vi "Min Buffer Size Test.vi"(7 "Fs (Hz)":dbl, 9 "Npts":i32) -> (15 "error out":errorcluster)   [LabVIEW 2015]
uses:
  <vilib>/DAQmx/write.llb/DAQmx Write (Digital Wfm 1Chan NSamp).vi
  <vilib>/DAQmx/write.llb/DAQmx Write (Analog 1D DBL 1Chan NSamp).vi
  <vilib>/DAQmx/create/channels.llb/DAQmx Create Channel (AO-Voltage-Basic).vi
  <vilib>/DAQmx/configure/timing.llb/DAQmx Timing (Sample Clock).vi
  <vilib>/DAQmx/miscellaneous.llb/DAQmx Fill In Error Info.vi
  <vilib>/DAQmx/create/channels.llb/DAQmx Create Channel (DO-Digital Output).vi
  <vilib>/Waveform/DWDTOps.llb/DWDT Boolean Array to Digital.vi
  <vilib>/Waveform/DWDTOps.llb/DWDT Uncompress Digital.vi
  <resource>/objmgr/daqmx.rc
panel:
  in  "stop":bool
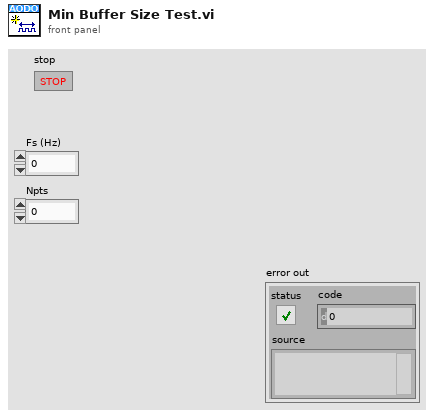
[diagram p1: front panel]
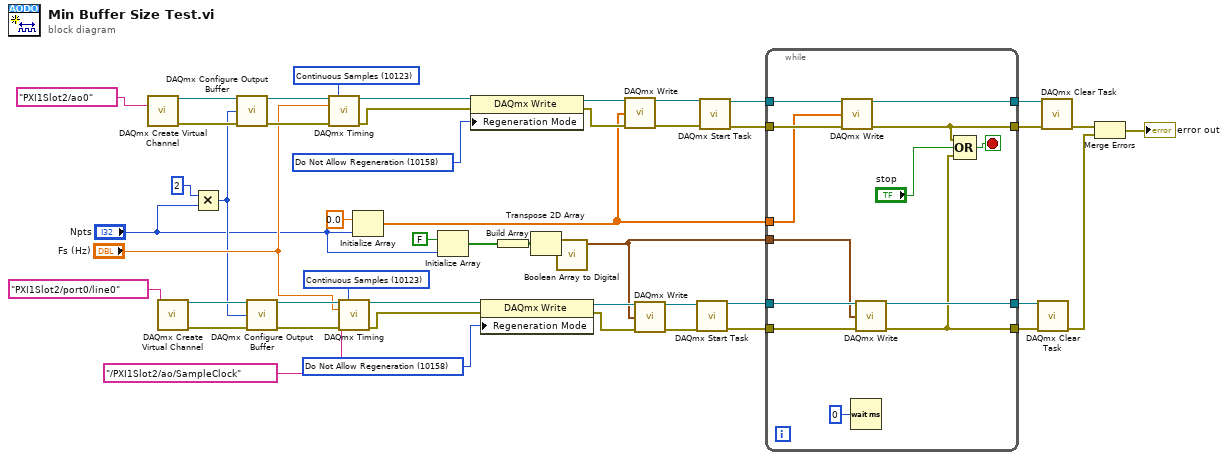
[diagram p0: block diagram]
diagram:
  w23 = 10158 items=["Allow Regeneration"=10097, "Do Not Allow Regeneration"=10158] ("RegenMode")
  w24 = 10123 items=["Finite Samples"=10178, "Continuous Samples"=10123, "Hardware Timed Single Point"=12522] ("sample mode")
  w43 = 10158 items=["Allow Regeneration"=10097, "Do Not Allow Regeneration"=10158] ("RegenMode")
  w44 = 10123 items=["Finite Samples"=10178, "Continuous Samples"=10123, "Hardware Timed Single Point"=12522] ("sample mode")
  n1 = call-poly <vilib>:"DAQmx Create Virtual Channel.vi"("physical channels"=tag "PXI1Slot2/ao0") -> ("task out"=w41:refnum<k21>, "error out"=w42:errorcluster)  [unwired: 13 in]
  n2 = call-poly <vilib>:"DAQmx Create Virtual Channel.vi"("lines"=tag "PXI1Slot2/port0/line0") -> ("task out"=w21:refnum<k21>, "error out"=w22:errorcluster)  [unwired: 13 in]
  n3 = Multiply(x=2 ("y"), y="Npts") -> (x*y=w15:i32)
  n4 = call <vilib>:"DAQmx Configure Output Buffer.vi"("task/channels in"=w41, "buffer size (in samples per channel)"=w15, "error in"=w42) -> ("task out"=w46:refnum<k21>, "error out"=w45:errorcluster)  [unwired: 11 in]
  n5 = call <vilib>:"DAQmx Configure Output Buffer.vi"("task/channels in"=w21, "buffer size (in samples per channel)"=w15, "error in"=w22) -> ("task out"=w26:refnum<k21>, "error out"=w25:errorcluster)  [unwired: 11 in]
  n6 = call-poly <vilib>:"DAQmx Timing.vi"("task/channels in"=w46, "sample mode"=w44, "rate"="Fs (Hz)", "error in"=w45) -> ("task out"=w48:refnum<k21>, "error out"=w47:errorcluster)  [unwired: 10 in]
  n7 = call-poly <vilib>:"DAQmx Timing.vi"("task/channels in"=w26, "sample mode"=w24, "rate"="Fs (Hz)", "source"=tag "/PXI1Slot2/ao/SampleClock", "error in"=w25) -> ("task out"=w28:refnum<k21>, "error out"=w27:errorcluster)  [unwired: 9 in]
  n8 = Initialize Array(0.0 ("element"), "Npts") -> (w32:dbl[])
  n9 = Initialize Array(FALSE, "Npts") -> (w12:bool[])
  n10 = property class="DAQmx Write"(reference=w48, error in=w47, "Regeneration Mode"=w43) -> (reference out=w39:refnum<k21>, error out=w38:errorcluster)
  n11 = property class="DAQmx Write"(reference=w28, error in=w27, "Regeneration Mode"=w23) -> (reference out=w20:refnum<k21>, error out=w19:errorcluster)
  n12 = Build Array(w12) -> (w11:bool[][])
  n13 = Transpose 2D Array(2D array=w11) -> (transposed array=w1:bool[][])
  n14 = call-poly <vilib>:"Boolean Array to Digital.vi"("boolean array"=w1) -> ("digital waveform"=w6:digitalwaveform)  [unwired: 9 in, 1 out]
  n15 = call-poly <vilib>:"DAQmx Write.vi"("task/channels in"=w39, "data"=w32, "error in"=w38) -> ("task out"=w36:refnum<k21>, "error out"=w35:errorcluster)  [unwired: 10 in, 1 out]
  n16 = call-poly <vilib>:"DAQmx Write.vi"("task/channels in"=w20, "data"=w6, "error in"=w19) -> ("task out"=w10:refnum<k21>, "error out"=w9:errorcluster)  [unwired: 10 in, 1 out]
  n17 = call <vilib>:"DAQmx Start Task.vi"("task/channels in"=w10, "error in"=w9) -> ("task out"=w8:refnum<k21>, "error out"=w7:errorcluster)  [unwired: 12 in]
  n18 = call <vilib>:"DAQmx Start Task.vi"("task/channels in"=w36, "error in"=w35) -> ("task out"=w33:refnum<k21>, "error out"=w34:errorcluster)  [unwired: 12 in]
  n19 = while {
    tunnel: w34 -> [w60]
    tunnel: w33 -> [w61]
    tunnel: w32 -> [w59]
    tunnel: [w57] -> w31
    tunnel: [w58] -> w30
    tunnel: w8 -> [w54]
    tunnel: w7 -> [w53]
    tunnel: w6 -> [w52]
    tunnel: [w51] -> w5
    tunnel: [w50] -> w4
    stop <- w55 stop-if-true
    n20 = call-poly <vilib>:"DAQmx Write.vi"("task/channels in"=w61, "data"=w59, "error in"=w60) -> ("task out"=w58:refnum<k21>, "error out"=w57:errorcluster)  [unwired: 10 in, 1 out]
    n21 = Wait (ms)(milliseconds to wait=u32 0) -> ()  [unwired: 1 out]
    n22 = call-poly <vilib>:"DAQmx Write.vi"("task/channels in"=w54, "data"=w52, "error in"=w53) -> ("task out"=w51:refnum<k21>, "error out"=w50:errorcluster)  [unwired: 10 in, 1 out]
    n23 = Compound Arithmetic op=OR(w57, "stop", w50) -> (w55:bool)
  }
  n24 = call <vilib>:"DAQmx Clear Task.vi"("task in"=w5, "error in"=w4) -> ("error out"=w2:errorcluster)  [unwired: 13 in]
  n25 = call <vilib>:"DAQmx Clear Task.vi"("task in"=w30, "error in"=w31) -> ("error out"=w29:errorcluster)  [unwired: 13 in]
  n26 = Merge Errors(w29, w2) -> (→"error out":errorcluster)
